vi "consumer.vi"(8 "error in (no error)":errorcluster, 10 "user event in":refnum<user-event>, 11 "Queue in":refnum<queue>) -> (0 "error out":errorcluster, 3 "user event out":refnum<user-event>)   [LabVIEW 2020]
uses:
  Type Defs/Message.ctl
  Type Defs/Local Data.ctl
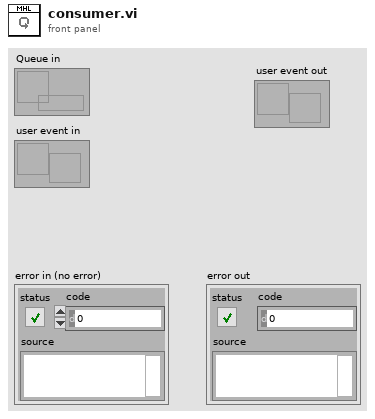
[diagram p1: front panel]
types:
  T1 = typedef "Local Data.ctl" = cluster{"Data":string}
  T2 = typedef "Message.ctl" = cluster{"Command":string, "Data":variant}
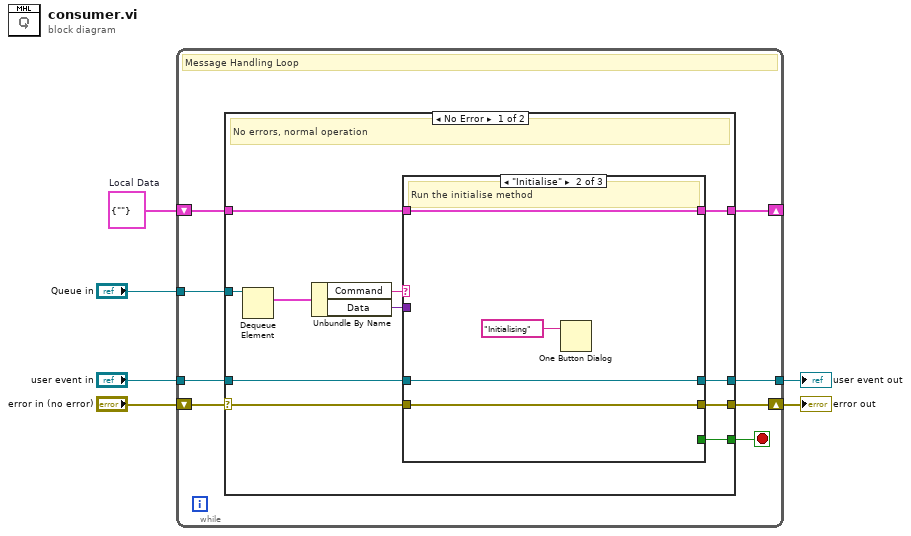
[diagram p0: block diagram]
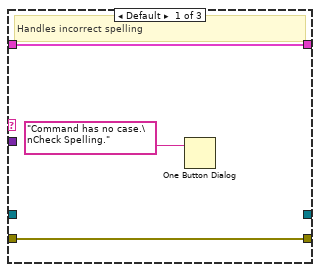
[diagram p2: hidden frame]
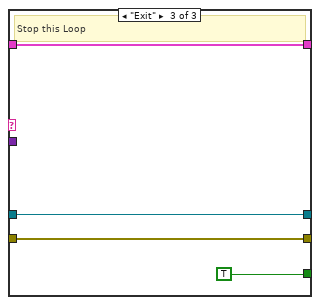
[diagram p3: hidden frame]
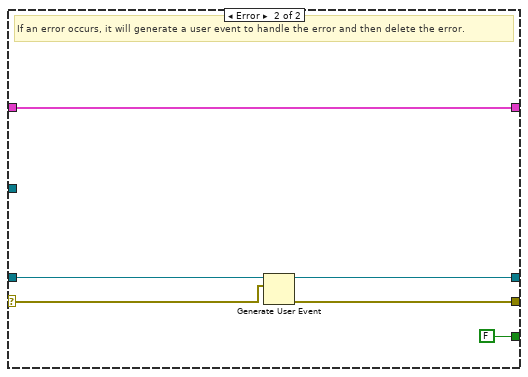
[diagram p4: hidden frame]
diagram:
  w6 = T1 {"Data"=""}  # Local Data
  n1 = while {
    tunnel: "user event in" -> [w13]
    tunnel: "Queue in" -> [w14]
    shift-right: [w12] -> w4
    shift-left: "error in (no error)" -> [w7]
    tunnel: [w10] -> w1
    shift-right: [w8] -> _
    shift-left: w6 -> [w9]
    stop <- w11 stop-if-true
    # "Message Handling Loop"
    n2 = case shown="No Error" w7 {
      selector: w7 -> [w15 w37]
      tunnel: w14 -> [w25 _]
      tunnel: w13 -> [w22 w40]
      tunnel: [w21 w39] -> w12
      tunnel: [w20 FALSE ("event data")] -> w11
      tunnel: [w18 w38] -> w10
      tunnel: w9 -> [w17 w42]
      tunnel: [w16 w42] -> w8
      frame No Error {
        # "No errors, normal operation"
        n3 = Dequeue Element(queue=w25) -> (element=w24:T2)  [unwired: 2 in, 3 out]
        n4 = Unbundle By Name "Unbundle By Name"(w24) -> ("Command"=w23:string, "Data"=w19:variant)
        n5 = case shown="\"Initialise\"" w23 {
          tunnel: w15 -> [w27 w32 w36]
          tunnel: w22 -> [_ w29 w35]
          tunnel: [w27 w32 w36] -> w21
          tunnel: [_ _ TRUE ("event data")] -> w20
          tunnel: w19 -> [_ _ _]
          tunnel: [_ w29 w35] -> w18
          tunnel: w17 -> [w26 w31 w33]
          tunnel: [w26 w31 w33] -> w16
          frame Default {
            # "Handles incorrect spelling"
            n6 = One Button Dialog(message="Command has no case.\nCheck Spelling.") -> ()  [unwired: 1 in, 1 out]
          }
          frame "Initialise" {
            # "Run the initialise method"
            n7 = One Button Dialog(message="Initialising") -> ()  [unwired: 1 in, 1 out]
          }
          frame "Exit" {
            # "Stop this Loop"
          }
        }
      }
      frame Error {
        # "If an error occurs, it will generate a user event to handle the error and then delete the error."
        n8 = Generate User Event(user event=w40, event data cluster=w37) -> (user event out=w38:refnum<user-event>, error out=w39:errorcluster)  [unwired: 2 in]
      }
    }
  }
  "error out" <- w4
  "user event out" <- w1
